vi "rsidr_core_global.vi"() -> ()   [LabVIEW 2020, in "Rohde&Schwarz RTx Oscilloscopes.lvlib"] (continued)
Models"="RTM|RTA", "Instrument Options"="", "Flags"=0, "Help"="Return the start time of the selected frame.\n\nAvailable Repeated Capabilities:\nSerialBus: SB1, SB2, SB3, SB4\r\n\nRemote-control command(s):\nBUS<b>:I2S:FRAMe<n>:STARt?"}, {"Level"=3, "Class Only"=FALSE, "Identifier"="RSRTX_ATTR_PROTOCOL_AUDIO_FRAME_STOP", "Descriptive Name"="Protocol Audio Frame Stop", "Data Type"=1, "Command"="BUS{SerialBus}:I2S:FRAM<Frame>:STOP?", "Access"=0, "Range Table"="", "Read Callback"="rsrtx_FormatAudioFrameRepCapReal_ReadCallback.vi", "Write Callback"="", "Supported Models"="RTM|RTA", "Instrument Options"="", "Flags"=0, "Help"="Return the stop time of the selected frame.\n\nAvailable Repeated Capabilities:\nSerialBus: SB1, SB2, SB3, SB4\r\n\nRemote-control command(s):\nBUS<b>:I2S:FRAMe<n>:STOP?"}, {"Level"=3, "Class Only"=FALSE, "Identifier"="RSRTX_ATTR_PROTOCOL_AUDIO_FRAME_LEFT_CHANNEL_STATUS", "Descriptive Name"="Protocol Audio Frame Left Channel Status", "Data Type"=0, "Command"="BUS{SerialBus}:I2S:FRAM<Frame>:LEFT:STAT?", "Access"=0, "Range Table"="rsrtx_rngAudioFrameStatus", "Read Callback"="rsrtx_FormatAudioFrameRepCapInt_ReadCallback.vi", "Write Callback"="", "Supported Models"="RTM|RTA", "Instrument Options"="", "Flags"=0, "Help"="Return the status of the left channel of the selected frame.\n\nAvailable Repeated Capabilities:\nSerialBus: SB1, SB2, SB3, SB4\r\n\nRemote-control command(s):\nBUS<b>:I2S:FRAMe<n>:LEFT:STATe?"}, {"Level"=3, "Class Only"=FALSE, "Identifier"="RSRTX_ATTR_PROTOCOL_AUDIO_FRAME_RIGHT_CHANNEL_STATUS", "Descriptive Name"="Protocol Audio Frame Right Channel Status", "Data Type"=0, "Command"="BUS{SerialBus}:I2S:FRAM<Frame>:RIGH:STAT?", "Access"=0, "Range Table"="rsrtx_rngAudioFrameStatus", "Read Callback"="rsrtx_FormatAudioFrameRepCapInt_ReadCallback.vi", "Write Callback"="", "Supported Models"="RTM|RTA", "Instrument Options"="", "Flags"=0, "Help"="Return the status of the right channel of the selected frame.\n\nAvailable Repeated Capabilities:\nSerialBus: SB1, SB2, SB3, SB4\r\n\nRemote-control command(s):\nBUS<b>:I2S:FRAMe<n>:RIGHt:STATe?"}, {"Level"=3, "Class Only"=FALSE, "Identifier"="RSRTX_ATTR_PROTOCOL_AUDIO_FRAME_LEFT_CHANNEL_VALUE", "Descriptive Name"="Protocol Audio Frame Left Channel Value", "Data Type"=1, "Command"="BUS{SerialBus}:I2S:FRAM<Frame>:LEFT:VAL?", "Access"=0, "Range Table"="", "Read Callback"="rsrtx_FormatAudioFrameRepCapReal_ReadCallback.vi", "Write Callback"="", "Supported Models"="RTM|RTA", "Instrument Options"="", "Flags"=0, "Help"="Return the data value of the left channel.\n\nAvailable Repeated Capabilities:\nSerialBus: SB1, SB2, SB3, SB4\r\n\nRemote-control command(s):\nBUS<b>:I2S:FRAMe<n>:LEFT:VALue?"}, {"Level"=3, "Class Only"=FALSE, "Identifier"="RSRTX_ATTR_PROTOCOL_AUDIO_FRAME_RIGHT_CHANNEL_VALUE", "Descriptive Name"="Protocol Audio Frame Right Channel Value", "Data Type"=1, "Command"="BUS{SerialBus}:I2S:FRAM<Frame>:RIGH:VAL?", "Access"=0, "Range Table"="", "Read Callback"="rsrtx_FormatAudioFrameRepCapReal_ReadCallback.vi", "Write Callback"="", "Supported Models"="RTM|RTA", "Instrument Options"="", "Flags"=0, "Help"="Return the data value of the right channel.\n\nAvailable Repeated Capabilities:\nSerialBus: SB1, SB2, SB3, SB4\r\n\nRemote-control command(s):\nBUS<b>:I2S:FRAMe<n>:RIGHt:VALue?"}, {"Level"=3, "Class Only"=TRUE, "Identifier"="", "Descriptive Name"="TDM Channel", "Data Type"=0, "Command"="", "Access"=0, "Range Table"="", "Read Callback"="", "Write Callback"="", "Supported Models"="", "Instrument Options"="", "Flags"=0, "Help"="This class contains attributes with TDMChannel repeated capability."}, {"Level"=4, "Class Only"=FALSE, "Identifier"="RSRTX_ATTR_PROTOCOL_AUDIO_FRAME_TDM_STATUS", "Descriptive Name"="Protocol Audio Frame TDM Status", "Data Type"=0, "Command"="BUS{SerialBus}:I2S:FRAM<Frame>:TDM{TDMChannel}:STAT?", "Access"=0, "Range Table"="rsrtx_rngAudioFrameStatus", "Read Callback"="rsrtx_FormatAudioFrameRepCapInt_ReadCallback.vi", "Write Callback"="", "Supported Models"="RTM|RTA", "Instrument Options"="", "Flags"=0, "Help"="Returns the state of the indicated channel of the selected frame.\n\nAvailable Repeated Capabilities:\nSerialBus: SB1, SB2, SB3, SB4\r\nTDMChannel: TDM0, TDM1, TDM2, TDM3, TDM4, TDM5, TDM6, TDM7, TDM8\r\n\nRemote-control command(s):\nBUS<b>:I2S:FRAMe<n>:TDM<o>:STATe?"}, {"Level"=4, "Class Only"=FALSE, "Identifier"="RSRTX_ATTR_PROTOCOL_AUDIO_FRAME_TDM_VALUE", "Descriptive Name"="Protocol Audio Frame TDM Value", "Data Type"=1, "Command"="BUS{SerialBus}:I2S:FRAM<Frame>:TDM{TDMChannel}:VAL?", "Access"=0, "Range Table"="", "Read Callback"="rsrtx_FormatAudioFrameRepCapReal_ReadCallback.vi", "Write Callback"="", "Supported Models"="RTM|RTA", "Instrument Options"="", "Flags"=0, "Help"="Return the data value of the indicated TDM channel.\n\nAvailable Repeated Capabilities:\nSerialBus: SB1, SB2, SB3, SB4\r\nTDMChannel: TDM0, TDM1, TDM2, TDM3, TDM4, TDM5, TDM6, TDM7, TDM8\r\n\nRemote-control command(s):\nBUS<b>:I2S:FRAMe<n>:TDM<o>:VALue?"}, {"Level"=3, "Class Only"=TRUE, "Identifier"="", "Descriptive Name"="Clock", "Data Type"=0, "Command"="", "Access"=0, "Range Table"="", "Read Callback"="", "Write Callback"="", "Supported Models"="", "Instrument Options"="", "Flags"=0, "Help"="Configures the clock line properties."}, {"Level"=4, "Class Only"=FALSE, "Identifier"="RSRTX_ATTR_PROTOCOL_AUDIO_CLOCK_SOURCE", "Descriptive Name"="Protocol Audio Clock Source", "Data Type"=0, "Command"="BUS{SerialBus}:I2S:CLOC:SOUR", "Access"=2, "Range Table"="rsrtx_rngAudioSource", "Read Callback"="", "Write Callback"="", "Supported Models"="RTM|RTA", "Instrument Options"="", "Flags"=0, "Help"="Selects the source of the waveform.\n\nAvailable Repeated Capabilities:\nSerialBus: SB1, SB2, SB3, SB4\r\n\nRemote-control command(s):\nBUS<b>:I2S:CLOCk:SOURce"}, {"Level"=4, "Class Only"=FALSE, "Identifier"="RSRTX_ATTR_PROTOCOL_AUDIO_CLOCK_THRESHOLD", "Descriptive Name"="Protocol Audio Clock Threshold", "Data Type"=1, "Command"="BUS{SerialBus}:I2S:CLOC:THR", "Access"=2, "Range Table"="", "Read Callback"="", "Write Callback"="", "Supported Models"="RTM|RTA", "Instrument Options"="", "Flags"=0, "Help"="Sets the threshold value for the clock line SCLK.\n\nAvailable Repeated Capabilities:\nSerialBus: SB1, SB2, SB3, SB4\r\n\nRemote-control command(s):\nBUS<b>:I2S:CLOCk:THReshold"}, {"Level"=4, "Class Only"=FALSE, "Identifier"="RSRTX_ATTR_PROTOCOL_AUDIO_CLOCK_POLARITY", "Descriptive Name"="Protocol Audio Clock Polarity", "Data Type"=0, "Command"="BUS{SerialBus}:I2S:CLOC:POL", "Access"=2, "Range Table"="rsrtx_rngAudioClockPolarity", "Read Callback"="", "Write Callback"="", "Supported Models"="RTM|RTA", "Instrument Options"="", "Flags"=0, "Help"="Selects line polarity.\n\nAvailable Repeated Capabilities:\nSerialBus: SB1, SB2, SB3, SB4\r\n\nRemote-control command(s):\nBUS<b>:I2S:CLOCk:POLarity"}, {"Level"=3, "Class Only"=TRUE, "Identifier"="", "Descriptive Name"="Word Select", "Data Type"=0, "Command"="", "Access"=0, "Range Table"="", "Read Callback"="", "Write Callback"="", "Supported Models"="", "Instrument Options"="", "Flags"=0, "Help"="Configures the word select line properties for I2S standard"}, {"Level"=4, "Class Only"=FALSE, "Identifier"="RSRTX_ATTR_PROTOCOL_AUDIO_WS_SOURCE", "Descriptive Name"="Protocol Audio WS Source", "Data Type"=0, "Command"="BUS{SerialBus}:I2S:WSEL:SOUR", "Access"=2, "Range Table"="rsrtx_rngAudioSource", "Read Callback"="", "Write Callback"="", "Supported Models"="RTM|RTA", "Instrument Options"="", "Flags"=0, "Help"="Selects the source of the word select line for I2S standard, left- und right-justified data formats, or the source of the frame synchronization pulse for TDM audio signals.\n\nAvailable Repeated Capabilities:\nSerialBus: SB1, SB2, SB3, SB4\r\n\nRemote-control command(s):\nBUS<b>:I2S:WSELect:SOURce"}, {"Level"=4, "Class Only"=FALSE, "Identifier"="RSRTX_ATTR_PROTOCOL_AUDIO_WS_THRESHOLD", "Descriptive Name"="Protocol Audio WS Threshold", "Data Type"=1, "Command"="BUS{SerialBus}:I2S:WSEL:THR", "Access"=2, "Range Table"="", "Read Callback"="", "Write Callback"="", "Supported Models"="RTM|RTA", "Instrument Options"="", "Flags"=0, "Help"="Sets the threshold value for the word select and FSYNC lines.\n\nAvailable Repeated Capabilities:\nSerialBus: SB1, SB2, SB3, SB4\r\n\nRemote-control command(s):\nBUS<b>:I2S:WSELect:THReshold"}, {"Level"=4, "Class Only"=FALSE, "Identifier"="RSRTX_ATTR_PROTOCOL_AUDIO_WS_POLARITY", "Descriptive Name"="Protocol Audio WS Polarity", "Data Type"=0, "Command"="BUS{SerialBus}:I2S:WSEL:POL", "Access"=2, "Range Table"="rsrtx_rngAudioWSPolarity", "Read Callback"="", "Write Callback"="", "Supported Models"="RTM|RTA", "Instrument Options"="", "Flags"=0, "Help"="Selects line polarity.\n\nAvailable Repeated Capabilities:\nSerialBus: SB1, SB2, SB3, SB4\r\n\nRemote-control command(s):\nBUS<b>:I2S:WSELect:POLarity"}, {"Level"=3, "Class Only"=TRUE, "Identifier"="", "Descriptive Name"="Data", "Data Type"=0, "Command"="", "Access"=0, "Range Table"="", "Read Callback"="", "Write Callback"="", "Supported Models"="", "Instrument Options"="", "Flags"=0, "Help"="Configures properties of the audio data line."}, {"Level"=4, "Class Only"=FALSE, "Identifier"="RSRTX_ATTR_PROTOCOL_AUDIO_DATA_SOURCE", "Descriptive Name"="Protocol Audio Data Source", "Data Type"=0, "Command"="BUS{SerialBus}:I2S:DATA:SOUR", "Access"=2, "Range Table"="rsrtx_rngAudioSource", "Read Callback"="", "Write Callback"="", "Supported Models"="RTM|RTA", "Instrument Options"="", "Flags"=0, "Help"="Selects the source of the audio data line.\n\nAvailable Repeated Capabilities:\nSerialBus: SB1, SB2, SB3, SB4\r\n\nRemote-control command(s):\nBUS<b>:I2S:DATA:SOURce"}, {"Level"=4, "Class Only"=FALSE, "Identifier"="RSRTX_ATTR_PROTOCOL_AUDIO_DATA_THRESHOLD", "Descriptive Name"="Protocol Audio Data Threshold", "Data Type"=1, "Command"="BUS{SerialBus}:I2S:DATA:THR", "Access"=2, "Range Table"="", "Read Callback"="", "Write Callback"="", "Supported Models"="RTM|RTA", "Instrument Options"="", "Flags"=0, "Help"="Sets the threshold value for the data line.\n\nAvailable Repeated Capabilities:\nSerialBus: SB1, SB2, SB3, SB4\r\n\nRemote-control command(s):\nBUS<b>:I2S:DATA:THReshold"}, {"Level"=4, "Class Only"=FALSE, "Identifier"="RSRTX_ATTR_PROTOCOL_AUDIO_DATA_POLARITY", "Descriptive Name"="Protocol Audio Data Polarity", "Data Type"=0, "Command"="BUS{SerialBus}:I2S:DATA:POL", "Access"=2, "Range Table"="rsrtx_rngProtocolSPIMISOPolarity", "Read Callback"="", "Write Callback"="", "Supported Models"="RTM|RTA", "Instrument Options"="", "Flags"=0, "Help"="Selects line polarity.\n\nAvailable Repeated Capabilities:\nSerialBus: SB1, SB2, SB3, SB4\r\n\nRemote-control command(s):\nBUS<b>:I2S:DATA:POLarity"}, {"Level"=3, "Class Only"=TRUE, "Identifier"="", "Descriptive Name"="Track Waveform", "Data Type"=0, "Command"="", "Access"=0, "Range Table"="", "Read Callback"="", "Write Callback"="", "Supported Models"="", "Instrument Options"="", "Flags"=0, "Help"="Selects Track Channel"}, {"Level"=4, "Class Only"=FALSE, "Identifier"="RSRTX_ATTR_PROTOCOL_AUDIO_TRACK_WAVEFORM_DISPLAY_MODE", "Descriptive Name"="Protocol Audio Track Waveform Display Mode", "Data Type"=0, "Command"="BUS{SerialBus}:I2S:DISP", "Access"=2, "Range Table"="rsrtx_rngTrackDisplayMode", "Read Callback"="", "Write Callback"="", "Supported Models"="RTM|RTA", "Instrument Options"="", "Flags"=0, "Help"="Defines how the decoded bus, the bit lines of the channels, and the track waveforms are displayed.\n\nAvailable Repeated Capabilities:\nSerialBus: SB1, SB2, SB3, SB4\r\n\nRemote-control command(s):\nBUS<b>:I2S:DISPlay"}, {"Level"=4, "Class Only"=FALSE, "Identifier"="RSRTX_ATTR_PROTOCOL_AUDIO_TRACK_WAVEFORM_LEFT_POSITION", "Descriptive Name"="Protocol Audio Track Waveform Left Position", "Data Type"=1, "Command"="BUS{SerialBus}:I2S:TRAC:LEFT:POS", "Access"=2, "Range Table"="", "Read Callback"="", "Write Callback"="", "Supported Models"="RTM|RTA", "Instrument Options"="", "Flags"=0, "Help"="Sets the vertical positiion of the track waveform for the left channel in divisions. The\ncommand is relevant for IS standard, left justified and right justified audio formats.s.\n\nAvailable Repeated Capabilities:\nSerialBus: SB1, SB2, SB3, SB4\r\n\nRemote-control command(s):\nBUS<b>:I2S:TRACk:LEFT:POSition"}, {"Level"=4, "Class Only"=FALSE, "Identifier"="RSRTX_ATTR_PROTOCOL_AUDIO_TRACK_WAVEFORM_LEFT_SCALE", "Descriptive Name"="Protocol Audio Track Waveform Left Scale", "Data Type"=1, "Command"="BUS{SerialBus}:I2S:TRAC:LEFT:SCAL", "Access"=2, "Range Table"="", "Read Callback"="", "Write Callback"="", "Supported Models"="RTM|RTA", "Instrument Options"="", "Flags"=0, "Help"="Sets the vertical scale of the track waveform for the left channel in bits per division.\n\nAvailable Repeated Capabilities:\nSerialBus: SB1, SB2, SB3, SB4\r\n\nRemote-control command(s):\nBUS<b>:I2S:TRACk:LEFT:SCALe"}, {"Level"=4, "Class Only"=FALSE, "Identifier"="RSRTX_ATTR_PROTOCOL_AUDIO_TRACK_WAVEFORM_RIGHT_POSITION", "Descriptive Name"="Protocol Audio Track Waveform Right Position", "Data Type"=1, "Command"="BUS{SerialBus}:I2S:TRAC:RIGH:POS", "Access"=2, "Range Table"="", "Read Callback"="", "Write Callback"="", "Supported Models"="RTM|RTA", "Instrument Options"="", "Flags"=0, "Help"="Sets the vertical positiion of the track waveform for the right channel in divisions. Relevant for IS standard, left justified and right justified audio formats.s.\n\nAvailable Repeated Capabilities:\nSerialBus: SB1, SB2, SB3, SB4\r\n\nRemote-control command(s):\nBUS<b>:I2S:TRACk:RIGHt:POSition"}, {"Level"=4, "Class Only"=FALSE, "Identifier"="RSRTX_ATTR_PROTOCOL_AUDIO_TRACK_WAVEFORM_RIGHT_SCALE", "Descriptive Name"="Protocol Audio Track Waveform Right Scale", "Data Type"=1, "Command"="BUS{SerialBus}:I2S:TRAC:RIGH:SCAL", "Access"=2, "Range Table"="", "Read Callback"="", "Write Callback"="", "Supported Models"="RTM|RTA", "Instrument Options"="", "Flags"=0, "Help"="Sets the vertical scale of the track waveform for the right channel in bits per division.\n\nAvailable Repeated Capabilities:\nSerialBus: SB1, SB2, SB3, SB4\r\n\nRemote-control command(s):\nBUS<b>:I2S:TRACk:RIGHt:SCALe"}, {"Level"=4, "Class Only"=FALSE, "Identifier"="RSRTX_ATTR_PROTOCOL_AUDIO_TRACK_WAVEFORM_SET_TO_DEFAULT", "Descriptive Name"="Protocol Audio Track Waveform Set To Default", "Data Type"=4, "Command"="BUS{SerialBus}:I2S:TRAC:SET:DEF", "Access"=1, "Range Table"="", "Read Callback"="", "Write Callback"="", "Supported Models"="RTM|RTA", "Instrument Options"="", "Flags"=0, "Help"="Sets all selected tracks to the middle of the display and scales them to full height of the display (8 dovisions). The track waveforms overlap.\n\nAvailable Repeated Capabilities:\nSerialBus: SB1, SB2, SB3, SB4\r\n\nRemote-control command(s):\nBUS<b>:I2S:TRACk:SET:DEFault"}, {"Level"=4, "Class Only"=FALSE, "Identifier"="RSRTX_ATTR_PROTOCOL_AUDIO_TRACK_WAVEFORM_SET_TO_SCREEN", "Descriptive Name"="Protocol Audio Track Waveform Set To Screen", "Data Type"=4, "Command"="BUS{SerialBus}:I2S:TRAC:SET:SCR", "Access"=1, "Range Table"="", "Read Callback"="", "Write Callback"="", "Supported Models"="RTM|RTA", "Instrument Options"="", "Flags"=0, "Help"="Arranges the selected tracks vertically, one above the other. The track waveforms do not overlap.\n\nAvailable Repeated Capabilities:\nSerialBus: SB1, SB2, SB3, SB4\r\n\nRemote-control command(s):\nBUS<b>:I2S:TRACk:SET:SCReen"}, {"Level"=4, "Class Only"=TRUE, "Identifier"="", "Descriptive Name"="Track Channel", "Data Type"=0, "Command"="", "Access"=0, "Range Table"="", "Read Callback"="", "Write Callback"="", "Supported Models"="", "Instrument Options"="", "Flags"=0, "Help"="Selects the track channel."}, {"Level"=5, "Class Only"=FALSE, "Identifier"="RSRTX_ATTR_PROTOCOL_AUDIO_TRACK_WAVEFORM_CHANNEL_ENABLED", "Descriptive Name"="Protocol Audio Track Waveform Channel Enabled", "Data Type"=3, "Command"="BUS{SerialBus}:I2S:TRAC:TDM{TDMChannel}:STAT", "Access"=2, "Range Table"="", "Read Callback"="", "Write Callback"="", "Supported Models"="RTM|RTA", "Instrument Options"="", "Flags"=0, "Help"="Defines if the indicated track waveform is visible on the display.\n\nAvailable Repeated Capabilities:\nSerialBus: SB1, SB2, SB3, SB4\r\nTDMChannel: TDM0, TDM1, TDM2, TDM3, TDM4, TDM5, TDM6, TDM7, TDM8\r\n\nRemote-control command(s):\nBUS<b>:I2S:TRACk:TDM<o>:STATe"}, {"Level"=5, "Class Only"=FALSE, "Identifier"="RSRTX_ATTR_PROTOCOL_AUDIO_TRACK_WAVEFORM_CHANNEL_POSITION", "Descriptive Name"="Protocol Audio Track Waveform Channel Position", "Data Type"=1, "Command"="BUS{SerialBus}:I2S:TRAC:TDM{TDMChannel}:POS", "Access"=2, "Range Table"="", "Read Callback"="", "Write Callback"="", "Supported Models"="RTM|RTA", "Instrument Options"="", "Flags"=0, "Help"="Sets the vertical positiion of the selected track waveform in divisions.\n\nAvailable Repeated Capabilities:\nSerialBus: SB1, SB2, SB3, SB4\r\nTDMChannel: TDM0, TDM1, TDM2, TDM3, TDM4, TDM5, TDM6, TDM7, TDM8\r\n\nRemote-control command(s):\nBUS<b>:I2S:TRACk:TDM<o>:POSition"}, {"Level"=5, "Class Only"=FALSE, "Identifier"="RSRTX_ATTR_PROTOCOL_AUDIO_TRACK_WAVEFORM_CHANNEL_SCALE", "Descriptive Name"="Protocol Audio Track Waveform Channel Scale", "Data Type"=1, "Command"="BUS{SerialBus}:I2S:TRAC:TDM{TDMChannel}:SCAL", "Access"=2, "Range Table"="", "Read Callback"="", "Write Callback"="", "Supported Models"="RTM|RTA", "Instrument Options"="", "Flags"=0, "Help"="Sets the vertical scale of the track waveform for the left channel in bits per division.\n\nAvailable Repeated Capabilities:\nSerialBus: SB1, SB2, SB3, SB4\r\nTDMChannel: TDM0, TDM1, TDM2, TDM3, TDM4, TDM5, TDM6, TDM7, TDM8\r\n\nRemote-control command(s):\nBUS<b>:I2S:TRACk:TDM<o>:SCALe"}, {"Level"=2, "Class Only"=TRUE, "Identifier"="", "Descriptive Name"="MILSTD", "Data Type"=0, "Command"="", "Access"=0, "Range Table"="", "Read Callback"="", "Write Callback"="", "Supported Models"="", "Instrument Options"="", "Flags"=0, "Help"="The MIL-STD-1553 specification defines the characteristics of a serial data bus originally designed for use in the military avionics. Nowadays it is also used in spacecraft on-board data handling."}, {"Level"=3, "Class Only"=FALSE, "Identifier"="RSRTX_ATTR_PROTOCOL_MILSTD_SOURCE", "Descriptive Name"="Protocol MILSTD Source", "Data Type"=0, "Command"="BUS{SerialBus}:MILS:SOUR", "Access"=2, "Range Table"="rsrtx_rngSource", "Read Callback"="", "Write Callback"="", "Supported Models"="RTM|RTA", "Instrument Options"="", "Flags"=0, "Help"="Sets the channel for the signal source.\n\nAvailable Repeated Capabilities:\nSerialBus: SB1, SB2, SB3, SB4\r\n\nRemote-control command(s):\nBUS<b>:MILStd:SOURce"}, {"Level"=3, "Class Only"=FALSE, "Identifier"="RSRTX_ATTR_PROTOCOL_MILSTD_POLARITY", "Descriptive Name"="Protocol MILSTD Polarity", "Data Type"=0, "Command"="BUS{SerialBus}:MILS:POL", "Access"=2, "Range Table"="rsrtx_rngPolarity", "Read Callback"="", "Write Callback"="", "Supported Models"="RTM|RTA", "Instrument Options"="", "Flags"=0, "Help"="Sets the polarity of the bus.\n\nAvailable Repeated Capabilities:\nSerialBus: SB1, SB2, SB3, SB4\r\n\nRemote-control command(s):\nBUS<b>:MILStd:POLarity"}, {"Level"=3, "Class Only"=FALSE, "Identifier"="RSRTX_ATTR_PROTOCOL_MILSTD_TRESHOLD_HIGH", "Descriptive Name"="Protocol MILSTD Treshold High", "Data Type"=1, "Command"="BUS{SerialBus}:MILS:THR:HIGH", "Access"=2, "Range Table"="", "Read Callback"="", "Write Callback"="", "Supported Models"="RTM|RTA", "Instrument Options"="", "Flags"=0, "Help"="Sets the upper threshold level of the signal.\n\nAvailable Repeated Capabilities:\nSerialBus: SB1, SB2, SB3, SB4\r\n\nRemote-control command(s):\nBUS<b>:MILStd:THReshold:HIGH"}, {"Level"=3, "Class Only"=FALSE, "Identifier"="RSRTX_ATTR_PROTOCOL_MILSTD_TRESHOLD_HLOW", "Descriptive Name"="Protocol MILSTD Treshold Low", "Data Type"=1, "Command"="BUS{SerialBus}:MILS:THR:LOW", "Access"=2, "Range Table"="", "Read Callback"="", "Write Callback"="", "Supported Models"="RTM|RTA", "Instrument Options"="", "Flags"=0, "Help"="Sets the lower threshold level of the signal.\n\nAvailable Repeated Capabilities:\nSerialBus: SB1, SB2, SB3, SB4\r\n\nRemote-control command(s):\nBUS<b>:MILStd:THReshold:LOW"}, {"Level"=3, "Class Only"=FALSE, "Identifier"="RSRTX_ATTR_PROTOCOL_MILSTD_TIMING", "Descriptive Name"="Protocol MILSTD Timing Deprecated", "Data Type"=1, "Command"="BUS{SerialBus}:MILS:RESP:MAX", "Access"=2, "Range Table"="", "Read Callback"="", "Write Callback"="", "Supported Models"="RTM|RTA", "Instrument Options"="", "Flags"=0, "Help"="Deprecated. Use RSRTX_ATTR_PROTOCOL_MILSTD_RESPONSE_TIME_MAXIMUM instead.\n\nAvailable Repeated Capabilities:\nSerialBus: SB1, SB2, SB3, SB4\r\n\nRemote-control command(s):\nBUS<b>:MILStd:RESPonsetime:MAXimum"}, {"Level"=3, "Class Only"=FALSE, "Identifier"="RSRTX_ATTR_PROTOCOL_MILSTD_INTER_MESSAGE_GAP_TIME_INFINITE", "Descriptive Name"="Protocol MILSTD Inter Message Gap Time Infinite", "Data Type"=3, "Command"="BUS{SerialBus}:MILS:IMGT:INF", "Access"=2, "Range Table"="", "Read Callback"="", "Write Callback"="", "Supported Models"="RTM|RTA", "Instrument Options"="", "Flags"=0, "Help"="Enables infinite Inter Message Gap Time.\n\nAvailable Repeated Capabilities:\nSerialBus: SB1, SB2, SB3, SB4\r\n\nRemote-control command(s):\nBUS<b>:MILStd:IMGTime:INFinite"}, {"Level"=3, "Class Only"=FALSE, "Identifier"="RSRTX_ATTR_PROTOCOL_MILSTD_INTER_MESSAGE_GAP_TIME_MINIMUM", "Descriptive Name"="Protocol MILSTD Inter Message Gap Time Minimum", "Data Type"=1, "Command"="BUS{SerialBus}:MILS:IMGT:MIN", "Access"=2, "Range Table"="", "Read Callback"="", "Write Callback"="", "Supported Models"="RTM|RTA", "Instrument Options"="", "Flags"=0, "Help"="Configures minimum Inter Message Gap Time.\n\nAvailable Repeated Capabilities:\nSerialBus: SB1, SB2, SB3, SB4\r\n\nRemote-control command(s):\nBUS<b>:MILStd:IMGTime:MINimum"}, {"Level"=3, "Class Only"=FALSE, "Identifier"="RSRTX_ATTR_PROTOCOL_MILSTD_INTER_MESSAGE_GAP_TIME_MAXIMUM", "Descriptive Name"="Protocol MILSTD Inter Message Gap Time Maximum", "Data Type"=1, "Command"="BUS{SerialBus}:MILS:IMGT:MAX", "Access"=2, "Range Table"="", "Read Callback"="", "Write Callback"="", "Supported Models"="RTM|RTA", "Instrument Options"="", "Flags"=0, "Help"="Configures maximum Inter Message Gap Time.\n\nAvailable Repeated Capabilities:\nSerialBus: SB1, SB2, SB3, SB4\r\n\nRemote-control command(s):\nBUS<b>:MILStd:IMGTime:MAXimum"}, {"Level"=3, "Class Only"=FALSE, "Identifier"="RSRTX_ATTR_PROTOCOL_MILSTD_RESPONSE_TIME_INFINITE", "Descriptive Name"="Protocol MILSTD Response Time Infinite", "Data Type"=3, "Command"="BUS{SerialBus}:MILS:RESP:INF", "Access"=2, "Range Table"="", "Read Callback"="", "Write Callback"="", "Supported Models"="RTM|RTA", "Instrument Options"="", "Flags"=0, "Help"="Enables infinite response time.\n\nAvailable Repeated Capabilities:\nSerialBus: SB1, SB2, SB3, SB4\r\n\nRemote-control command(s):\nBUS<b>:MILStd:RESPonsetime:INFinite"}, {"Level"=3, "Class Only"=FALSE, "Identifier"="RSRTX_ATTR_PROTOCOL_MILSTD_RESPONSE_TIME_MINIMUM", "Descriptive Name"="Protocol MILSTD Response Time Minimum", "Data Type"=1, "Command"="BUS{SerialBus}:MILS:RESP:MIN", "Access"=2, "Range Table"="", "Read Callback"="", "Write Callback"="", "Supported Models"="RTM|RTA", "Instrument Options"="", "Flags"=0, "Help"="Configures minimum response time.\n\nAvailable Repeated Capabilities:\nSerialBus: SB1, SB2, SB3, SB4\r\n\nRemote-control command(s):\nBUS<b>:MILStd:RESPonsetime:MINimum"}, {"Level"=3, "Class Only"=FALSE, "Identifier"="RSRTX_ATTR_PROTOCOL_MILSTD_RESPONSE_TIME_MAXIMUM", "Descriptive Name"="Protocol MILSTD Response Time Maximum", "Data Type"=1, "Command"="BUS{SerialBus}:MILS:RESP:MAX", "Access"=2, "Range Table"="", "Read Callback"="", "Write Callback"="", "Supported Models"="RTM|RTA", "Instrument Options"="", "Flags"=0, "Help"="Configures maximum response time.\n\nAvailable Repeated Capabilities:\nSerialBus: SB1, SB2, SB3, SB4\r\n\nRemote-control command(s):\nBUS<b>:MILStd:RESPonsetime:MAXimum"}, {"Level"=3, "Class Only"=TRUE, "Identifier"="", "Descriptive Name"="Word Results", "Data Type"=0, "Command"="", "Access"=0, "Range Table"="", "Read Callback"="", "Write Callback"="", "Supported Models"="", "Instrument Options"="", "Flags"=0, "Help"="Word results."}, {"Level"=4, "Class Only"=FALSE, "Identifier"="RSRTX_ATTR_PROTOCOL_MILSTD_WORD_COUNT", "Descriptive Name"="Protocol MILSTD Word Count", "Data Type"=0, "Command"="BUS{SerialBus}:MILS:WCO?", "Access"=0, "Range Table"="", "Read Callback"="", "Write Callback"="", "Supported Models"="RTM|RTA", "Instrument Options"="", "Flags"=0, "Help"="Returns the number of received words.\n\nAvailable Repeated Capabilities:\nSerialBus: SB1, SB2, SB3, SB4\r\n\nRemote-control command(s):\nBUS<b>:MILStd:WCOunt?"}, {"Level"=4, "Class Only"=FALSE, "Identifier"="RSRTX_ATTR_PROTOCOL_MILSTD_SELECTED_WORD", "Descriptive Name"="Protocol MILSTD Selected Word", "Data Type"=0, "Command"="", "Access"=2, "Range Table"="", "Read Callback"="", "Write Callback"="", "Supported Models"="", "Instrument Options"="", "Flags"=0, "Help"="Sets selector repeated capability Word.\n\nAvailable Repeated Capabilities:\nNone\n\nRemote-control command(s):\n"}, {"Level"=4, "Class Only"=FALSE, "Identifier"="RSRTX_ATTR_PROTOCOL_MILSTD_WORD_START", "Descriptive Name"="Protocol MILSTD Word Start", "Data Type"=1, "Command"="BUS{SerialBus}:MILS:WORD<Word>:STAR?", "Access"=0, "Range Table"="", "Read Callback"="rsrtx_FormatMILSTDWordRepCapReal_ReadCallback.vi", "Write Callback"="", "Supported Models"="RTM|RTA", "Instrument Options"="", "Flags"=0, "Help"="Returns the start time of the specified word.\n\nAvailable Repeated Capabilities:\nSerialBus: SB1, SB2, SB3, SB4\r\n\nRemote-control command(s):\nBUS<b>:MILStd:WORD<n>:STARt?"}, {"Level"=4, "Class Only"=FALSE, "Identifier"="RSRTX_ATTR_PROTOCOL_MILSTD_WORD_STOP", "Descriptive Name"="Protocol MILSTD Word Stop", "Data Type"=1, "Command"="BUS{SerialBus}:MILS:WORD<Word>:STOP?", "Access"=0, "Range Table"="", "Read Callback"="rsrtx_FormatMILSTDWordRepCapReal_ReadCallback.vi", "Write Callback"="", "Supported Models"="RTM|RTA", "Instrument Options"="", "Flags"=0, "Help"="Returns the stop time of the specified word.\n\nAvailable Repeated Capabilities:\nSerialBus: SB1, SB2, SB3, SB4\r\n\nRemote-control command(s):\nBUS<b>:MILStd:WORD<n>:STOP?"}, {"Level"=4, "Class Only"=FALSE, "Identifier"="RSRTX_ATTR_PROTOCOL_MILSTD_WORD_STATUS", "Descriptive Name"="Protocol MILSTD Word Status", "Data Type"=0, "Command"="BUS{SerialBus}:MILS:WORD<Word>:STAT?", "Access"=0, "Range Table"="rsrtx_rngMILSTDStatus", "Read Callback"="rsrtx_FormatMILSTDWordRepCapInt_ReadCallback.vi", "Write Callback"="", "Supported Models"="RTM|RTA", "Instrument Options"="", "Flags"=0, "Help"="For a status word returns the value and if there are errors.\n\nAvailable Repeated Capabilities:\nSerialBus: SB1, SB2, SB3, SB4\r\n\nRemote-control command(s):\nBUS<b>:MILStd:WORD<n>:STATus?"}, {"Level"=4, "Class Only"=FALSE, "Identifier"="RSRTX_ATTR_PROTOCOL_MILSTD_WORD_TRANSMISSION_DIRECTION", "Descriptive Name"="Protocol MILSTD Word Transmission Direction", "Data Type"=0, "Command"="BUS{SerialBus}:MILS:WORD<Word>:TRM?", "Access"=0, "Range Table"="rsrtx_rngMILSTDDirection", "Read Callback"="rsrtx_FormatMILSTDWordRepCapInt_ReadCallback.vi", "Write Callback"="", "Supported Models"="RTM|RTA", "Instrument Options"="", "Flags"=0, "Help"="Returns the transmission direction of the specified word.\n\nAvailable Repeated Capabilities:\nSerialBus: SB1, SB2, SB3, SB4\r\n\nRemote-control command(s):\nBUS<b>:MILStd:WORD<n>:TRMode?"}, {"Level"=4, "Class Only"=FALSE, "Identifier"="RSRTX_ATTR_PROTOCOL_MILSTD_WORD_TYPE", "Descriptive Name"="Protocol MILSTD Word Type", "Data Type"=0, "Command"="BUS{SerialBus}:MILS:WORD<Word>:TYPE?", "Access"=0, "Range Table"="rsrtx_rngMILSTDType", "Read Callback"="rsrtx_FormatMILSTDWordRepCapInt_ReadCallback.vi", "Write Callback"="", "Supported Models"="RTM|RTA", "Instrument Options"="", "Flags"=0, "Help"="Returns the type of word of the specified word.\n\nAvailable Repeated Capabilities:\nSerialBus: SB1, SB2, SB3, SB4\r\n\nRemote-control command(s):\nBUS<b>:MILStd:WORD<n>:TYPE?"}, {"Level"=4, "Class Only"=FALSE, "Identifier"="RSRTX_ATTR_PROTOCOL_MILSTD_WORD_PARITY", "Descriptive Name"="Protocol MILSTD Word Parity", "Data Type"=0, "Command"="BUS{SerialBus}:MILS:WORD<Word>:PAR?", "Access"=0, "Range Table"="", "Read Callback"="rsrtx_FormatMILSTDWordRepCapInt_ReadCallback.vi", "Write Callback"="", "Supported Models"="RTM|RTA", "Instrument Options"="", "Flags"=0, "Help"="Returns the parity of the specified word.\n\nAvailable Repeated Capabilities:\nSerialBus: SB1, SB2, SB3, SB4\r\n\nRemote-control command(s):\nBUS<b>:MILStd:WORD<n>:PARity?"}, {"Level"=4, "Class Only"=FALSE, "Identifier"="RSRTX_ATTR_PROTOCOL_MILSTD_WORD_RESPONSE_TIME", "Descriptive Name"="Protocol MILSTD Word Response Time", "Data Type"=1, "Command"="BUS{SerialBus}:MILS:WORD<Word>:RTIM?", "Access"=0, "Range Table"="", "Read Callback"="rsrtx_FormatMILSTDWordRepCapReal_ReadCallback.vi", "Write Callback"="", "Supported Models"="RTM|RTA", "Instrument Options"="", "Flags"=0, "Help"="Return the response time of the specified word.\n\nAvailable Repeated Capabilities:\nSerialBus: SB1, SB2, SB3, SB4\r\n\nRemote-control command(s):\nBUS<b>:MILStd:WORD<n>:RTIMe?"}, {"Level"=4, "Class Only"=FALSE, "Identifier"="RSRTX_ATTR_PROTOCOL_MILSTD_WORD_VALUE", "Descriptive Name"="Protocol MILSTD Word Value", "Data Type"=1, "Command"="BUS{SerialBus}:MILS:WORD<Word>:DATA?", "Access"=0, "Range Table"="", "Read Callback"="rsrtx_FormatMILSTDWordRepCapReal_ReadCallback.vi", "Write Callback"="", "Supported Models"="RTM|RTA", "Instrument Options"="", "Flags"=0, "Help"="Returns the value of the specified data word.\n\nAvailable Repeated Capabilities:\nSerialBus: SB1, SB2, SB3, SB4\r\n\nRemote-control command(s):\nBUS<b>:MILStd:WORD<n>:DATA?"}, {"Level"=4, "Class Only"=FALSE, "Identifier"="RSRTX_ATTR_PROTOCOL_MILSTD_WORD_INTERMESSAGE_GATE_TIME", "Descriptive Name"="Protocol MILSTD Word Intermessage Gate Time", "Data Type"=1, "Command"="BUS{SerialBus}:MILS:WORD<Word>:IMGT?", "Access"=0, "Range Table"="", "Read Callback"="rsrtx_FormatMILSTDWordRepCapReal_ReadCallback.vi", "Write Callback"="", "Supported Models"="RTM|RTA", "Instrument Options"="", "Flags"=0, "Help"="Returns the intermessage gate time of the specified word.\n\nAvailable Repeated Capabilities:\nSerialBus: SB1, SB2, SB3, SB4\r\n\nRemote-control command(s):\nBUS<b>:MILStd:WORD<n>:IMGTime?"}, {"Level"=4, "Class Only"=TRUE, "Identifier"="", "Descriptive Name"="Command", "Data Type"=0, "Command"="", "Access"=0, "Range Table"="", "Read Callback"="", "Write Callback"="", "Supported Models"="", "Instrument Options"="", "Flags"=0, "Help"="Command word attributes."}, {"Level"=5, "Class Only"=FALSE, "Identifier"="RSRTX_ATTR_PROTOCOL_MILSTD_COMMAND_WORD_COUNT", "Descriptive Name"="Protocol MILSTD Command Word Count", "Data Type"=0, "Command"="BUS{SerialBus}:MILS:WORD<Word>:COMM:WCO?", "Access"=0, "Range Table"="", "Read Callback"="rsrtx_FormatMILSTDWordRepCapInt_ReadCallback.vi", "Write Callback"="", "Supported Models"="RTM|RTA", "Instrument Options"="", "Flags"=0, "Help"="For a command word, returns the word count.\n\nAvailable Repeated Capabilities:\nSerialBus: SB1, SB2, SB3, SB4\r\n\nRemote-control command(s):\nBUS<b>:MILStd:WORD<n>:COMMand:WCOunt?"}, {"Level"=5, "Class Only"=FALSE, "Identifier"="RSRTX_ATTR_PROTOCOL_MILSTD_COMMAND_WORD_MODE_CODE_TYPE", "Descriptive Name"="Protocol MILSTD Command Word Mode Code Type", "Data Type"=0, "Command"="BUS{SerialBus}:MILS:WORD<Word>:COMM:MCOD:CODE?", "Access"=0, "Range Table"="rsrtx_rngMILSTDCodeType", "Read Callback"="rsrtx_FormatMILSTDWordRepCapInt_ReadCallback.vi", "Write Callback"="", "Supported Models"="RTM|RTA", "Instrument Options"="", "Flags"=0, "Help"="For the sepcified command word, returns the type of mode code.\n\nAvailable Repeated Capabilities:\nSerialBus: SB1, SB2, SB3, SB4\r\n\nRemote-control command(s):\nBUS<b>:MILStd:WORD<n>:COMMand:MCODe:CODE?"}, {"Level"=5, "Class Only"=FALSE, "Identifier"="RSRTX_ATTR_PROTOCOL_MILSTD_COMMAND_WORD_MODE_CODE_VALUE", "Descriptive Name"="Protocol MILSTD Command Word Mode Code Value", "Data Type"=1, "Command"="BUS{SerialBus}:MILS:WORD<Word>:COMM:MCOD:VAL?", "Access"=0, "Range Table"="", "Read Callback"="rsrtx_FormatMILSTDWordRepCapReal_ReadCallback.vi", "Write Callback"="", "Supported Models"="RTM|RTA", "Instrument Options"="", "Flags"=0, "Help"="For the specified command word, returns the value of the mode code.\n\nAvailable Repeated Capabilities:\nSerialBus: SB1, SB2, SB3, SB4\r\n\nRemote-control command(s):\nBUS<b>:MILStd:WORD<n>:COMMand:MCODe:VALue?"}, {"Level"=5, "Class Only"=FALSE, "Identifier"="RSRTX_ATTR_PROTOCOL_MILSTD_COMMAND_WORD_RT_ADDRESS", "Descriptive Name"="Protocol MILSTD Command Word RT Address", "Data Type"=2, "Command"="BUS{SerialBus}:MILS:WORD<Word>:COMM:RTAD?", "Access"=0, "Range Table"="", "Read Callback"="rsrtx_FormatMILSTDWordRepCapString_ReadCallback.vi", "Write Callback"="", "Supported Models"="RTM|RTA", "Instrument Options"="", "Flags"=0, "Help"="Returns the RT address of the specified word.\n\nAvailable Repeated Capabilities:\nSerialBus: SB1, SB2, SB3, SB4\r\n\nRemote-control command(s):\nBUS<b>:MILStd:WORD<n>:COMMand:RTADdress?"}, {"Level"=5, "Class Only"=FALSE, "Identifier"="RSRTX_ATTR_PROTOCOL_MILSTD_COMMAND_WORD_SUB_ADDRESS", "Descriptive Name"="Protocol MILSTD Command Word Sub Address", "Data Type"=2, "Command"="BUS{SerialBus}:MILS:WORD<Word>:COMM:SADD?", "Access"=0, "Range Table"="", "Read Callback"="rsrtx_FormatMILSTDWordRepCapString_ReadCallback.vi", "Write Callback"="", "Supported Models"="RTM|RTA", "Instrument Options"="", "Flags"=0, "Help"="For a command word, returns the subaddress of the specified word.\n\nAvailable Repeated Capabilities:\nSerialBus: SB1, SB2, SB3, SB4\r\n\nRemote-control command(s):\nBUS<b>:MILStd:WORD<n>:COMMand:SADDress?"}, {"Level"=4, "Class Only"=TRUE, "Identifier"="", "Descriptive Name"="Bit Status", "Data Type"=0, "Command"="", "Access"=0, "Range Table"="", "Read Callback"="", "Write Callback"="", "Supported Models"="", "Instrument Options"="", "Flags"=0, "Help"="Bit status attributes."}, {"Level"=5, "Class Only"=FALSE, "Identifier"="RSRTX_ATTR_PROTOCOL_MILSTD_WORD_RECEIVED_BIT_STATUS", "Descriptive Name"="Protocol MILSTD Word Received Bit Status", "Data Type"=0, "Command"="BUS{SerialBus}:MILS:WORD<Word>:STAT:BCR?", "Access"=0, "Range Table"="", "Read Callback"="rsrtx_FormatMILSTDWordRepCapInt_ReadCallback.vi", "Write Callback"="", "Supported Models"="RTM|RTA", "Instrument Options"="", "Flags"=0, "Help"="Returns the state of the broadcast command received bit of the specified status word.\n\nAvailable Repeated Capabilities:\nSerialBus: SB1, SB2, SB3, SB4\r\n\nRemote-control command(s):\nBUS<b>:MILStd:WORD<n>:STATus:BCReceived?"}, {"Level"=5, "Class Only"=FALSE, "Identifier"="RSRTX_ATTR_PROTOCOL_MILSTD_WORD_BUSY_BIT_STATUS", "Descriptive Name"="Protocol MILSTD Word Busy Bit Status", "Data Type"=0, "Command"="BUS{SerialBus}:MILS:WORD<Word>:STAT:BUSY?", "Access"=0, "Range Table"="", "Read Callback"="rsrtx_FormatMILSTDWordRepCapInt_ReadCallback.vi", "Write Callback"="", "Supported Models"="RTM|RTA", "Instrument Options"="", "Flags"=0, "Help"="Returns the state of the busy bit of the specified status word.\n\nAvailable Repeated Capabilities:\nSerialBus: SB1, SB2, SB3, SB4\r\n\nRemote-control command(s):\nBUS<b>:MILStd:WORD<n>:STATus:BUSY?"}, {"Level"=5, "Class Only"=FALSE, "Identifier"="RSRTX_ATTR_PROTOCOL_MILSTD_WORD_BUS_CONTROL_BIT_STATUS", "Descriptive Name"="Protocol MILSTD Word Bus Control Bit Status", "Data Type"=0, "Command"="BUS{SerialBus}:MILS:WORD<Word>:STAT:DBC?", "Access"=0, "Range Table"="", "Read Callback"="rsrtx_FormatMILSTDWordRepCapInt_ReadCallback.vi", "Write Callback"="", "Supported Models"="RTM|RTA", "Instrument Options"="", "Flags"=0, "Help"="Returns the state of the dynamic bus control bit of the specified status word.\n\nAvailable Repeated Capabilities:\nSerialBus: SB1, SB2, SB3, SB4\r\n\nRemote-control command(s):\nBUS<b>:MILStd:WORD<n>:STATus:DBCaccept?"}, {"Level"=5, "Class Only"=FALSE, "Identifier"="RSRTX_ATTR_PROTOCOL_MILSTD_WORD_INSTRUMENTATION_BIT_STATUS", "Descriptive Name"="Protocol MILSTD Word Instrumentation Bit Status", "Data Type"=0, "Command"="BUS{SerialBus}:MILS:WORD<Word>:STAT:INST?", "Access"=0, "Range Table"="", "Read Callback"="rsrtx_FormatMILSTDWordRepCapInt_ReadCallback.vi", "Write Callback"="", "Supported Models"="RTM|RTA", "Instrument Options"="", "Flags"=0, "Help"="Returns the state of the instrumentation bit of the specified status word.\n\nAvailable Repeated Capabilities:\nSerialBus: SB1, SB2, SB3, SB4\r\n\nRemote-control command(s):\nBUS<b>:MILStd:WORD<n>:STATus:INSTrument?"}, {"Level"=5, "Class Only"=FALSE, "Identifier"="RSRTX_ATTR_PROTOCOL_MILSTD_WORD_MESSAGE_ERROR_BIT_STATUS", "Descriptive Name"="Protocol MILSTD Word Message Error Bit Status", "Data Type"=0, "Command"="BUS{SerialBus}:MILS:WORD<Word>:STAT:MERR?", "Access"=0, "Range Table"="", "Read Callback"="rsrtx_FormatMILSTDWordRepCapInt_ReadCallback.vi", "Write Callback"="", "Supported Models"="RTM|RTA", "Instrument Options"="", "Flags"=0, "Help"="Returns the state of the message error bit of the specified status word.\n\nAvailable Repeated Capabilities:\nSerialBus: SB1, SB2, SB3, SB4\r\n\nRemote-control command(s):\nBUS<b>:MILStd:WORD<n>:STATus:MERRor?"}, {"Level"=5, "Class Only"=FALSE, "Identifier"="RSRTX_ATTR_PROTOCOL_MILSTD_WORD_STATUS_RT_ADDRESS", "Descriptive Name"="Protocol MILSTD Word Status RT Address", "Data Type"=2, "Command"="BUS{SerialBus}:MILS:WORD<Word>:STAT:RTAD?", "Access"=0, "Range Table"="", "Read Callback"="rsrtx_FormatMILSTDWordRepCapString_ReadCallback.vi", "Write Callback"="", "Supported Models"="RTM|RTA", "Instrument Options"="", "Flags"=0, "Help"="Returns the RT address of the specified status word.\n\nAvailable Repeated Capabilities:\nSerialBus: SB1, SB2, SB3, SB4\r\n\nRemote-control command(s):\nBUS<b>:MILStd:WORD<n>:STATus:RTADdress?"}, {"Level"=5, "Class Only"=FALSE, "Identifier"="RSRTX_ATTR_PROTOCOL_MILSTD_WORD_SUBSYSTEM_BIT_STATUS", "Descriptive Name"="Protocol MILSTD Word Subsystem Bit Status", "Data Type"=0, "Command"="BUS{SerialBus}:MILS:WORD<Word>:STAT:SUBS?", "Access"=0, "Range Table"="", "Read Callback"="rsrtx_FormatMILSTDWordRepCapInt_ReadCallback.vi", "Write Callback"="", "Supported Models"="RTM|RTA", "Instrument Options"="", "Flags"=0, "Help"="Returns the state of the subsystem bit of the specified status word.\n\nAvailable Repeated Capabilities:\nSerialBus: SB1, SB2, SB3, SB4\r\n\nRemote-control command(s):\nBUS<b>:MILStd:WORD<n>:STATus:SUBSystem?"}, {"Level"=5, "Class Only"=FALSE, "Identifier"="RSRTX_ATTR_PROTOCOL_MILSTD_WORD_TERMINAL_BIT_STATUS", "Descriptive Name"="Protocol MILSTD Word Terminal Bit Status", "Data Type"=0, "Command"="BUS{SerialBus}:MILS:WORD<Word>:STAT:TERM?", "Access"=0, "Range Table"="", "Read Callback"="rsrtx_FormatMILSTDWordRepCapInt_ReadCallback.vi", "Write Callback"="", "Supported Models"="RTM|RTA", "Instrument Options"="", "Flags"=0, "Help"="Returns the state of the terminal flag bit of the specified status word.\n\nAvailable Repeated Capabilities:\nSerialBus: SB1, SB2, SB3, SB4\r\n\nRemote-control command(s):\nBUS<b>:MILStd:WORD<n>:STATus:TERMinal?"}, {"Level"=5, "Class Only"=FALSE, "Identifier"="RSRTX_ATTR_PROTOCOL_MILSTD_WORD_SERVICE_REQUEST_BIT_STATUS", "Descriptive Name"="Protocol MILSTD Word Service Request Bit Status", "Data Type"=0, "Command"="BUS{SerialBus}:MILS:WORD<Word>:STAT:SREQ?", "Access"=0, "Range Table"="", "Read Callback"="rsrtx_FormatMILSTDWordRepCapInt_ReadCallback.vi", "Write Callback"="", "Supported Models"="RTM|RTA", "Instrument Options"="", "Flags"=0, "Help"="Returns the state of the service request bit of the specified word.\n\nAvailable Repeated Capabilities:\nSerialBus: SB1, SB2, SB3, SB4\r\n\nRemote-control command(s):\nBUS<b>:MILStd:WORD<n>:STATus:SREQuest?"}, 
